vi "CAL-Compute Group Delay.vi"(0 "user path":path, 11 "error in (no error)":errorcluster) -> (8 "group delay (ms)":dbl, 15 "error out":errorcluster)   [LabVIEW 2020]
uses:
  <vilib>/Analysis/6fits.llb/Curve Fitting Criteria.ctl
  <vilib>/Analysis/NI_AALPro.lvlib
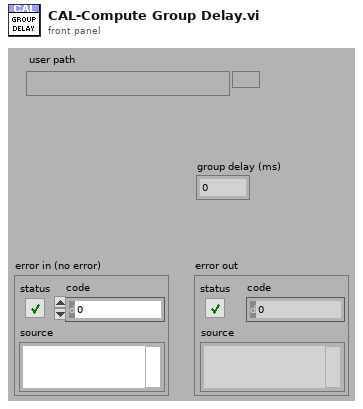
[diagram p1: front panel]
types:
  T1 = typedef "NI_AALPro.lvlib/Curve Fitting Criteria.ctl" = u16
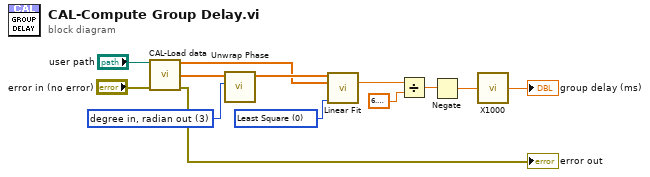
[diagram p0: block diagram]
diagram:
  w9 = T1 0 items=["Least Square", "Least Absolute Residual", "Bisquare"] ("method")
  w10 = 3 items=["radian in, radian out", "radian in, degree out", "degree in, degree out", "degree in, radian out"] ("phase unit")
  n1 = call "CAL-Load data.vi"("user path"="user path", "error in (no error)"="error in (no error)") -> ("Frequency (Hz)"=w7:dbl[], "Phase"=w11:dbl[], "error out"=→"error out":errorcluster)  [unwired: 6 in, 5 out]
  n2 = call <vilib>:"Unwrap Phase.vi"("phase unit"=w10, "Phase"=w11) -> ("Unwrapped Phase"=w8:dbl[])  [unwired: 8 in, 1 out]
  n3 = call <vilib>:"Linear Fit.vi"("Y"=w8, "X"=w7, "method"=w9) -> ("slope"=w6:dbl)  [unwired: 8 in, 4 out]
  n4 = Divide(x=w6, y=6.283185307179586) -> (x/y=w2:dbl)
  n5 = Negate(x=w2) -> (-x=w5:dbl)
  n6 = call "X1000.vi"("X"=w5) -> ("X/1000"=→"group delay (ms)":dbl)
